vi "MPExxx_get_ext_ctrl.vi"(0 "VISA session":refnum<visa-resource-name>, 1 "error in (no error)":errorcluster) -> (2 "dup VISA session":refnum<visa-resource-name>, 3 "External Control State":string, 4 "error out":errorcluster)   [LabVIEW 2012]
doc: "This VI form retrieves the external control setting.\n\nValues:\n0 - External control off\n1 - External control on"
panel:
  # "MAGNA-POWER"
  # "Electronics"
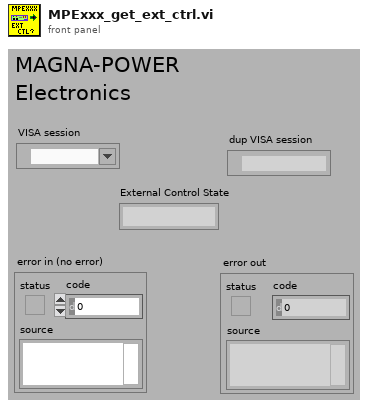
[diagram p1: front panel]
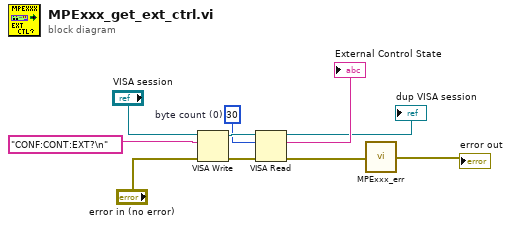
[diagram p0: block diagram]
diagram:
  w8 = u32 30  # byte count (0)
  n1 = VISA Write(VISA resource name="VISA session", write buffer="CONF:CONT:EXT?\n", error in (no error)="error in (no error)") -> (VISA resource name out=w9:refnum<visa-resource-name>, error out=w7:errorcluster)  [unwired: 1 out]
  n2 = VISA Read(VISA resource name=w9, byte count=w8, error in (no error)=w7) -> (VISA resource name out=→"dup VISA session":refnum<visa-resource-name>, read buffer=→"External Control State":string, error out=w5:errorcluster)  [unwired: 1 out]
  n3 = call "MPExxx_err.vi"("error in (no error)"=w5) -> ("error out"=→"error out":errorcluster)
